vi "Initiate Updates.vi"(8 "error in (no error)":errorcluster, 11 "MediatorBusMonitor In":refnum<class "MediatorBusMonitor.lvclass">) -> (0 "error out":errorcluster, 3 "MediatorBusMonitor Out":refnum<class "MediatorBusMonitor.lvclass">)   [LabVIEW 2017, in "Mediator.lvlib" / "MediatorBusMonitor.lvclass"]
doc: "<License>\nCopyright © 2017 Composed Systems, LLC | All rights reserved\nwww.composed.io\n\nAuthor: Ethan Stern <ethan.stern@composed.io>\n\nThis software is provided \"AS IS\" WITHOUT WARRANTIES, either express or implied, AND IS FOR EDUCATIONAL PURPOSES ONLY.\n</License>"
uses:
  MediatorBusMonitor.lvclass
  IMediator/IMediatorBusMonitor/MediatorBusMonitor/IMediatorBusMonitor.lvclass
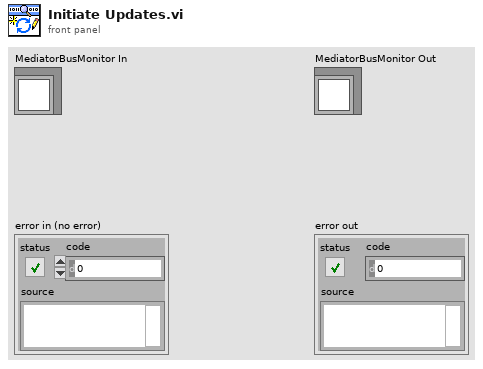
[diagram p1: front panel]
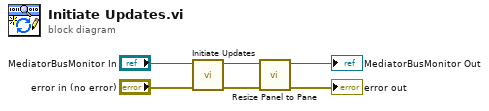
[diagram p0: block diagram]
diagram:
  n1 = call-parent "Initiate Updates.vi"("error in (no error)"="error in (no error)", "IViewable In"="MediatorBusMonitor In") -> ("error out"=w2:errorcluster, "IViewable Out"=w6:refnum<class "MediatorBusMonitor.lvclass">)  [unwired: 8 in]
  n2 = call-dynamic "Resize Panel to Pane.vi"("error in (no error)"=w2, "MediatorBusMonitor In"=w6) -> ("error out"=→"error out":errorcluster, "MediatorBusMonitor Out"=→"MediatorBusMonitor Out":refnum<class "MediatorBusMonitor.lvclass">)  [unwired: 8 in]
